vi "CLI.gh.vi"(8 "error in (no error)":errorcluster, 10 "Command":string, 11 "Git in":refnum<class "Git.lvclass">) -> (0 "error out":errorcluster, 1 "standard error":string, 2 "standard output":string, 3 "Git out":refnum<class "Git.lvclass">, 4 "return code":i32)   [LabVIEW 2019, in "Git.lvclass"]
uses:
  Git.lvclass
  Git.lvclass/Git.ctl
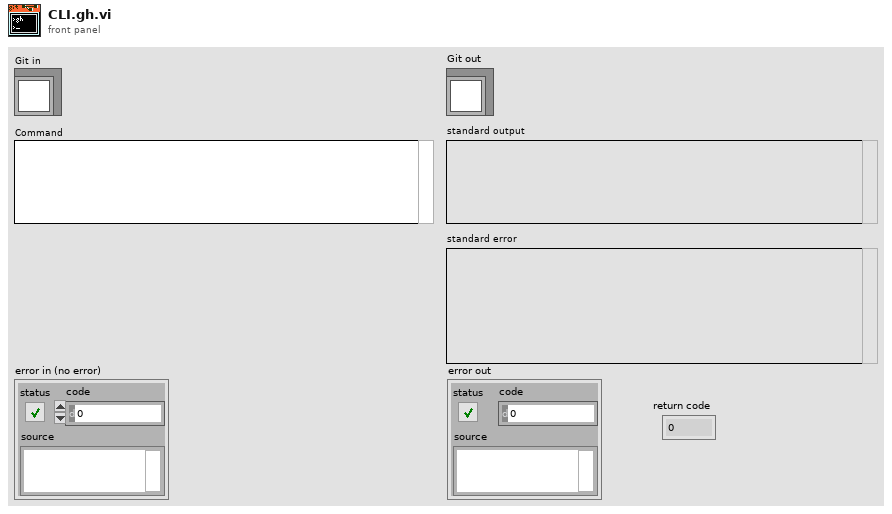
[diagram p1: front panel]
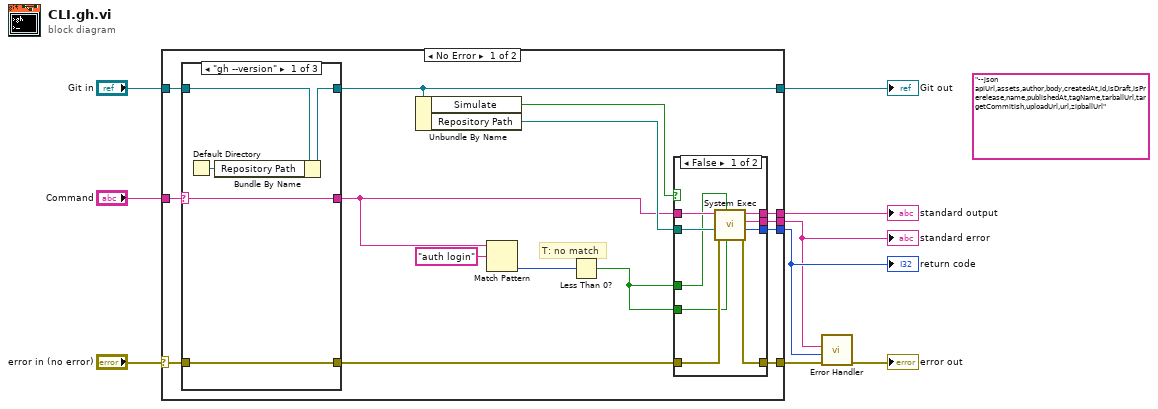
[diagram p0: block diagram]
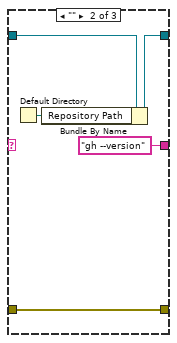
[diagram p2: hidden frame]
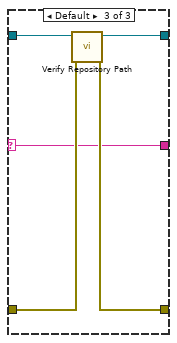
[diagram p3: hidden frame]
diagram:
  (unwired) "--json apiUrl,assets,author,body,createdAt,id,isDraft,isPrerelease,name,publishedAt,tagName,tarballUrl,targetCommitish,uploadUrl,url,zipballUrl"
  n1 = case shown="No Error" "error in (no error)" {
    selector: "error in (no error)" -> [w16 w52]
    tunnel: [w24 _] -> w6
    tunnel: [w23 w52] -> w4
    tunnel: [w22 _] -> w1
    tunnel: [w21 _] -> w2
    tunnel: "Git in" -> [w20 w51]
    tunnel: [w18 w51] -> w8
    tunnel: "Command" -> [w11 _]
    frame No Error {
      # "T: no match"
      n2 = case shown="\"gh --version\"" w11 {
        selector: w11 -> [w28 _ w35]
        tunnel: w20 -> [w25 w31 w39]
        tunnel: [w27 w33 w38] -> w19
        tunnel: [w26 w32 w37] -> w18
        tunnel: w16 -> [w27 w33 w36]
        tunnel: [w28 "gh --version" w35] -> w10
        frame "gh --version" {
          n3 = Default Directory() -> (w29:path)
          n4 = Bundle By Name(cluster=w25, "Repository Path"=w29) -> (w26:refnum<class "Git.lvclass">)
        }
        frame "" {
          n5 = Default Directory() -> (w34:path)
          n6 = Bundle By Name(cluster=w31, "Repository Path"=w34) -> (w32:refnum<class "Git.lvclass">)
        }
        frame Default {
          n7 = call "Verify Repository Path.vi"("error in (no error)"=w36, "Git in"=w39) -> ("error out"=w38:errorcluster, "Git out"=w37:refnum<class "Git.lvclass">)  [unwired: 8 in]
        }
      }
      n8 = Unbundle By Name(w18) -> ("Simulate"=w15:bool, "Repository Path"=w17:path)
      n9 = Match Pattern(string=w10, regular expression="auth login") -> (offset past match=w12:i32)  [unwired: 1 in, 3 out]
      n10 = Less Than 0?(x=w12) -> (x < 0?=w14:bool)
      n11 = case shown="False" w15 {
        tunnel: [w48 w50] -> w24
        tunnel: [w42 w49] -> w23
        tunnel: [w47 _] -> w22
        tunnel: [w46 _] -> w21
        tunnel: w19 -> [w45 w49]
        tunnel: w10 -> [w44 w50]
        tunnel: w17 -> [w43 _]
        tunnel: w14 -> [w41 _]
        tunnel: w14 -> [w40 _]
        frame False {
          n12 = call <vilib>:"System Exec.vi"("run minimized? (F)"=w41, "wait until completion? (T)"=w40, "error in (no error)"=w45, "working directory"=w43, "command line"=w44) -> ("error out"=w42:errorcluster, "return code"=w46:i32, "standard error"=w47:string, "standard output"=w48:string)  [unwired: 3 in]
        }
        frame True {
        }
      }
    }
    frame Error {
    }
  }
  "standard output" <- w6
  "standard error" <- w1
  "return code" <- w2
  "Git out" <- w8
  n13 = call "Error Handler.vi"("error in (no error)"=w4, "return code"=w2, "standard error"=w1) -> ("error out"=→"error out":errorcluster)  [unwired: 8 in]
